vi "task5.vi"() -> ()   [LabVIEW 2015]
uses:
  <vilib>/httpClient/POSTBuffer.vi
  <vilib>/httpClient/LabVIEWHTTPClient.lvlib
panel:
  in  "data":string
  out "body 3":string
  out "headers 3":string
  in  "Get":bool
  out "body 2":string
  out "headers 2":string
  in  "PUT":bool
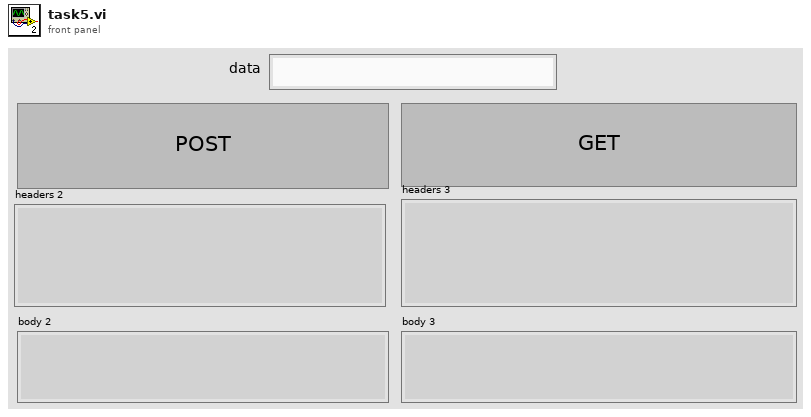
[diagram p1: front panel]
types:
  T1 = typedef "LabVIEWHTTPClient.lvlib/ClientHandle.ctl" = refnum<k1>
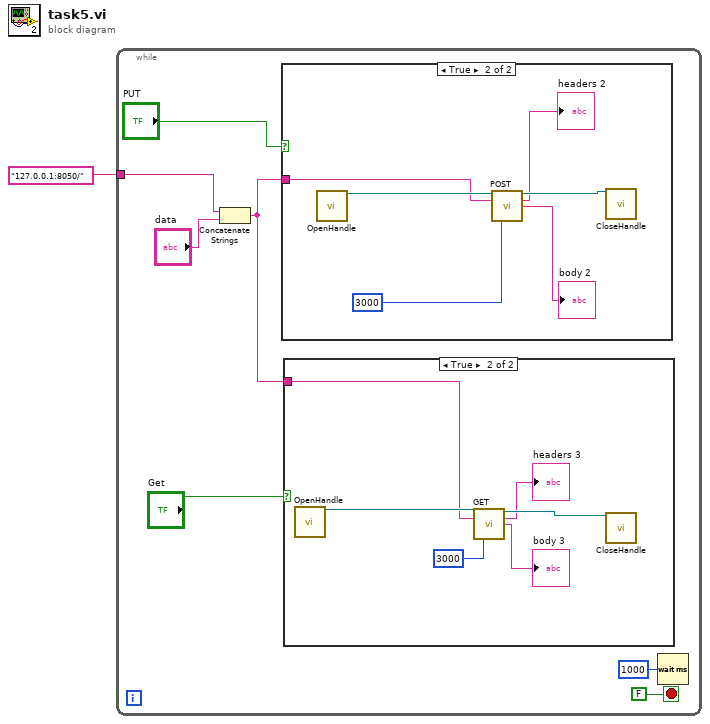
[diagram p0: block diagram]
diagram:
  n1 = while {
    tunnel: "127.0.0.1:8050/" ("url") -> [w3]
    stop <- FALSE stop-if-true
    n2 = Concatenate Strings(w3, "data") -> (w2:string)
    n3 = case shown="True" "PUT" {
      tunnel: w2 -> [_ w15]
      frame False {
      }
      frame True {
        n4 = call <vilib>:"OpenHandle.vi"() -> ("client handle out"=w18:T1)  [unwired: 14 in, 1 out]
        n5 = call-poly <vilib>:"POST.vi"("client handle"=w18, "url"=w15, "timeout (10000)"=3000) -> ("client handle out"=w20:T1, "headers"=→"headers 2":string, "body"=→"body 2":string)  [unwired: 9 in, 1 out]
        n6 = call <vilib>:"CloseHandle.vi"("client handle"=w20) -> ()  [unwired: 14 in, 1 out]
      }
    }
    n7 = case shown="True" "Get" {
      tunnel: w2 -> [_ w9]
      frame False {
      }
      frame True {
        n8 = call <vilib>:"OpenHandle.vi"() -> ("client handle out"=w10:T1)  [unwired: 14 in, 1 out]
        n9 = call <vilib>:"GET.vi"("client handle"=w10, "url"=w9, "timeout (10000)"=3000) -> ("client handle out"=w14:T1, "headers"=→"headers 3":string, "body"=→"body 3":string)  [unwired: 9 in, 1 out]
        n10 = call <vilib>:"CloseHandle.vi"("client handle"=w14) -> ()  [unwired: 14 in, 1 out]
      }
    }
    n11 = Wait (ms)(milliseconds to wait=u32 1000) -> ()  [unwired: 1 out]
  }
